vi "1BS3HD BinaryRecord.vi"(4 "Record":bool, 9 "File name":path, 10 "wfm":i16[][](array[numeric]), 11 "Chan params":T1) -> ()   [LabVIEW 2013]
panel:
  out "error out":errorcluster
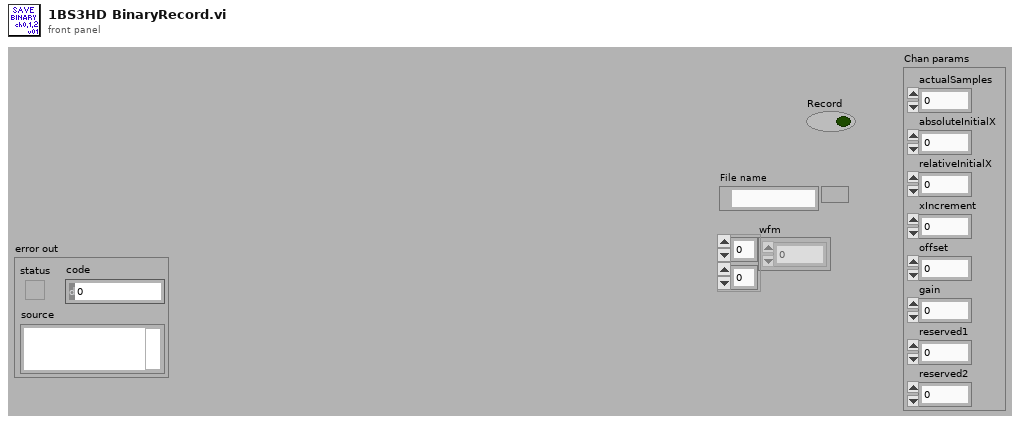
[diagram p1: front panel]
types:
  T1 = cluster{"actualSamples":i32, "absoluteInitialX":dbl, "relativeInitialX":dbl, "xIncrement":dbl, "offset":dbl, "gain":dbl, "reserved1":dbl, "reserved2":dbl}
  T2 = enum16{"open", "replace", "create", "open or create", "replace or create", "replace or create with confirmation"}
  T3 = enum16{"big-endian, network order", "native, host order", "little-endian"}
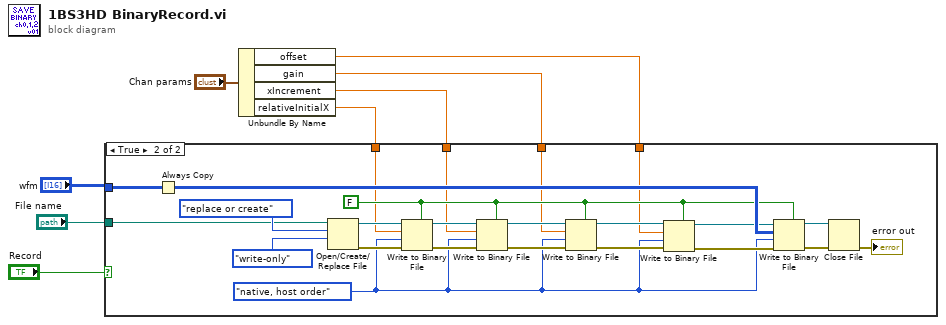
[diagram p0: block diagram]
diagram:
  n1 = Unbundle By Name("Chan params") -> ("offset"=w2:dbl, "gain"=w3:dbl, "xIncrement"=w4:dbl, "relativeInitialX"=w5:dbl)
  n2 = case shown="True" "Record" {
    tunnel: "wfm" -> [_ w10]
    tunnel: w5 -> [_ w14]
    tunnel: w4 -> [_ w13]
    tunnel: w3 -> [_ w12]
    tunnel: w2 -> [_ w11]
    tunnel: "File name" -> [_ w9]
    frame False {
    }
    frame True {
      w16 = FALSE ("prepend array or string size? (T)")
      w17 = T3."native, host order" ("byte order (0:big-endian, network order)")
      n3 = Always Copy(1:w10) -> (0:w30:i16[][])
      n4 = Open/Create/Replace File(file path (use dialog)=w9, operation (0:open)=T2."replace or create", access (0:read/write)=enum16{"read/write", "read-only", "write-only"}."write-only") -> (refnum out=w29:refnum<file>, error out=w28:errorcluster)  [unwired: 1 in, 3 out]
      n5 = Write to Binary File(file (use dialog)=w29, data=w14, error in=w28, 5:w16, 9:w17) -> (refnum out=w27:refnum<file>, error out=w26:errorcluster)  [unwired: 2 out]
      n6 = Write to Binary File(file (use dialog)=w27, data=w13, error in=w26, 5:w16, 9:w17) -> (refnum out=w25:refnum<file>, error out=w21:errorcluster)  [unwired: 2 out]
      n7 = Write to Binary File(file (use dialog)=w25, data=w12, error in=w21, 5:w16, 9:w17) -> (refnum out=w24:refnum<file>, error out=w20:errorcluster)  [unwired: 2 out]
      n8 = Write to Binary File(file (use dialog)=w24, data=w11, error in=w20, 5:w16, 9:w17) -> (refnum out=w23:refnum<file>, error out=w19:errorcluster)  [unwired: 2 out]
      n9 = Write to Binary File(file (use dialog)=w23, data=w30, error in=w19, 5:w16, 9:w17) -> (refnum out=w22:refnum<file>, error out=w18:errorcluster)  [unwired: 2 out]
      n10 = Close File(refnum=w22, error in=w18) -> (error out=→"error out":errorcluster)  [unwired: 1 out]
    }
  }
